vi "Begin.vi"() -> (0 "error out":errorcluster)   [LabVIEW 2023]
doc: "Called before other user functions, this VI is expected to open initial I/O refnums, load in file data, and do all program initialization. Notice that the <B>error out</B> terminal is simply used for data flow. Wiring it to other structures or subVIs ensures that this VI runs first."
uses:
  <vilib>/Rock Robotics/WPI/DriverStation/WPI_DriverStationRobotMode2.ctl
  Robot Global Data.vi
  <vilib>/Rock Robotics/Network Tables/NT Write String Array.vi
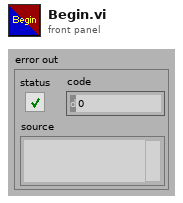
[diagram p1: front panel]
types:
  T1 = typedef "WPI_DriverStationRobotMode2.ctl" = enum16{"Autonomous Disabled", "Autonomous Enabled", "Teleop Disabled", "Teleop Enabled", "Disconnected", "Finish", "Test Disabled", "Test Enabled", "Emergency Stopped"}
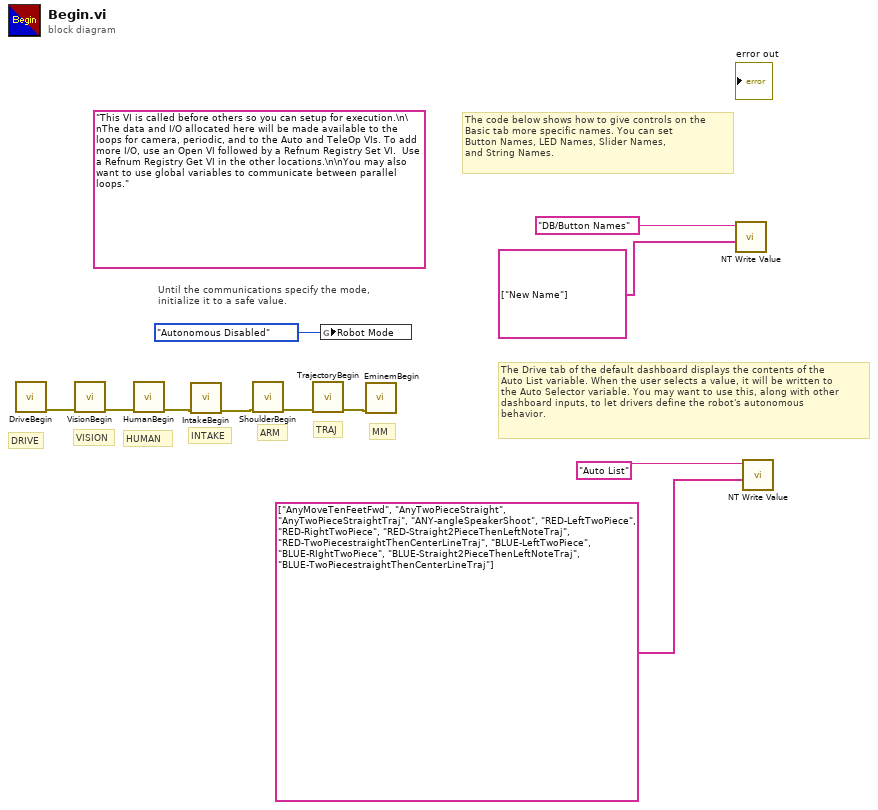
[diagram p0: block diagram]
diagram:
  (unwired) "This VI is called before others so you can setup for execution.\n\nThe data and I/O allocated here will be made available to the loops for camera, periodic, and to the Auto and TeleOp VIs. To add more I/O, use an Open VI followed by a Refnum Registry Set VI.  Use a Refnum Registry Get VI in the other locations.\n\nYou may also want to use global variables to communicate between parallel loops."
  # "MM"
  # "TRAJ"
  # "INTAKE"
  # "HUMAN"
  # "VISION"
  # "DRIVE"
  # "ARM"
  # "The Drive tab of the default dashboard displays the contents of the\nAuto List variable. When the user selects a value, it will be written to\nthe Auto Selector variable. You may want to use this, along with other\ndashboard inputs, to let drivers define the robot's autonomous\nbehavior."
  # "The code below shows how to give controls on the\nBasic tab more specific names. You can set\nButton Names, LED Names, Slider Names,\nand String Names."
  # "Until the communications specify the mode,\ninitialize it to a safe value."
  n1 = call "DriveBegin.vi"() -> ("error out"=w6:errorcluster)  [unwired: 11 in]
  n2 = call "VisionBegin.vi"("error in (no error)"=w6) -> ("error out"=w5:errorcluster)  [unwired: 10 in]
  n3 = call "HumanBegin.vi"("error in (no error)"=w5) -> ("error out"=w3:errorcluster)  [unwired: 10 in]
  n4 = call "IntakeBegin.vi"("error in (no error)"=w3) -> ("error out"=w2:errorcluster)  [unwired: 10 in]
  n5 = call "ShoulderBegin.vi"("error in (no error)"=w2) -> ("error out"=w4:errorcluster)  [unwired: 10 in]
  n6 = call "TrajectoryBegin.vi"("error in (no error)"=w4) -> ("error out"=w1:errorcluster)  [unwired: 10 in]
  n7 = global write "Robot Global Data.vi" "Robot Mode"(WPI_DriverStationRobotMode2."Autonomous Disabled" ("Robot Mode")) -> ()
  n8 = call "EminemBegin.vi"("error in (no error)"=w1) -> ()  [unwired: 8 in, 1 out]
  n9 = call-poly <vilib>:"NT Write Value.vi"("value"=string[] ["New Name"], "name"="DB/Button Names" ("Name")) -> ()  [unwired: 9 in, 1 out]
  n10 = call-poly <vilib>:"NT Write Value.vi"("value"=string[] ["AnyMoveTenFeetFwd", "AnyTwoPieceStraight", "AnyTwoPieceStraightTraj", "ANY-angleSpeakerShoot", "RED-LeftTwoPiece", "RED-RightTwoPiece", "RED-Straight2PieceThenLeftNoteTraj", "RED-TwoPiecestraightThenCenterLineTraj", "BLUE-LeftTwoPiece", "BLUE-RIghtTwoPiece", "BLUE-Straight2PieceThenLeftNoteTraj", "BLUE-TwoPiecestraightThenCenterLineTraj"] ("String Array"), "name"="Auto List" ("Name")) -> ()  [unwired: 9 in, 1 out]
